vi "pp2_updateSessionInfoCLEAR.vi"(10 "Session info In":T1 {"T Jump%" format="%.3g"; "N Jump%" format="%.3g"; "G Jump%" format="%.3g"}) -> (2 "Session info Out":T1 {"T Jump%" format="%.3g"; "N Jump%" format="%.3g"; "G Jump%" format="%.3g"})   [LabVIEW 2013]
uses:
  pp3_CTL_SessionInfo.ctl
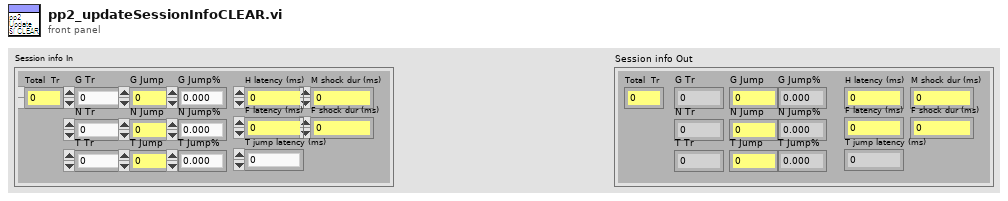
[diagram p1: front panel]
types:
  T1 = typedef "pp3_CTL_SessionInfo.ctl" = cluster{"Total  Tr":u32, "G Tr":u32, "G Jump":u32, "G Jump%":dbl, "N Tr":u32, "N Jump":u32, "N Jump%":dbl, "T Tr":u32, "T Jump":u32, "T Jump%":dbl, "M shock dur (ms)":dbl, "F shock dur (ms)":dbl, "H latency (ms)":dbl, "F latency (ms)":dbl, "T jump latency (ms)":dbl}
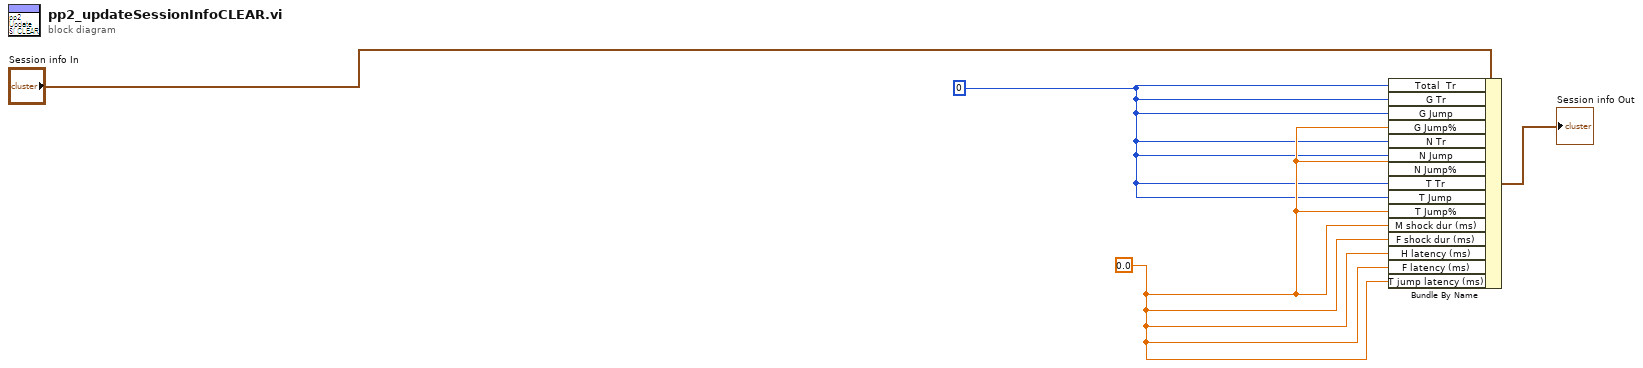
[diagram p0: block diagram]
diagram:
  w1 = u32 0 ("index")
  w2 = 0.0 ("index")
  n1 = Bundle By Name(cluster="Session info In", "Total  Tr"=w1, "G Tr"=w1, "G Jump"=w1, "G Jump%"=w2, "N Tr"=w1, "N Jump"=w1, "N Jump%"=w2, "T Tr"=w1, "T Jump"=w1, "T Jump%"=w2, "M shock dur (ms)"=w2, "F shock dur (ms)"=w2, "H latency (ms)"=w2, "F latency (ms)"=w2, "T jump latency (ms)"=w2) -> (→"Session info Out":T1)
